vi "JNC Im.vi"(8 "error in (no error)":errorcluster, 10 "Im":u8 format="%04b", 11 "TD4 in":refnum<class "TD4.lvclass">) -> (0 "error out":errorcluster, 3 "TD4 out":refnum<class "TD4.lvclass">)   [LabVIEW 2025, in "TD4.lvclass"]
uses:
  TD4.lvclass
  TD4.lvclass/TD4.ctl
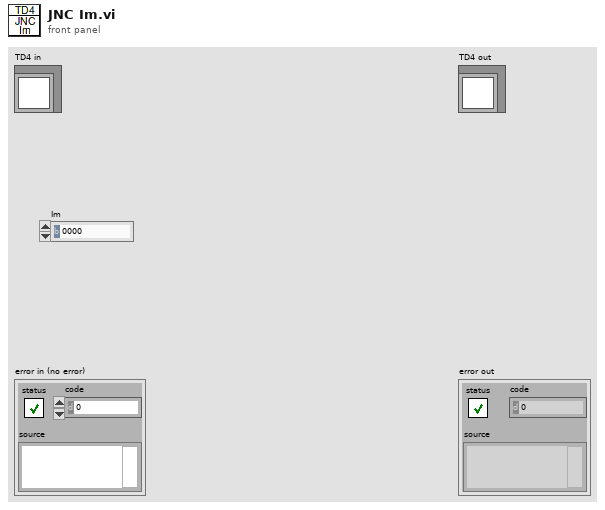
[diagram p1: front panel]
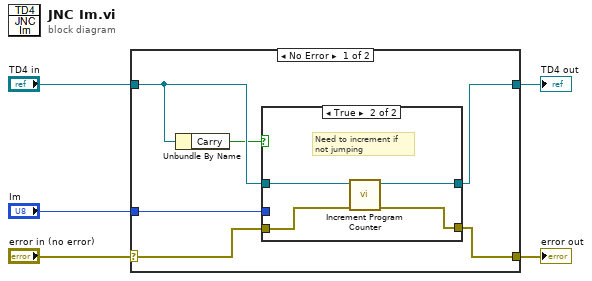
[diagram p0: block diagram]
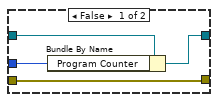
[diagram p2: hidden frame]
diagram:
  n1 = case shown="No Error" "error in (no error)" {
    selector: "error in (no error)" -> [w7 w20]
    tunnel: [w6 w20] -> w4
    tunnel: [w9 w21] -> w2
    tunnel: "TD4 in" -> [w10 w21]
    tunnel: "Im" -> [w11 _]
    frame No Error {
      n2 = Unbundle By Name(w10) -> ("Carry"=w8:bool)
      n3 = case shown="True" w8 {
        tunnel: w11 -> [w15 _]
        tunnel: w10 -> [w14 w19]
        tunnel: [w13 w18] -> w9
        tunnel: w7 -> [w12 w17]
        tunnel: [w12 w16] -> w6
        frame False {
          n4 = Bundle By Name(cluster=w14, "Program Counter"=w15) -> (w13:refnum<class "TD4.lvclass">)
        }
        frame True {
          # "Need to increment if \nnot jumping"
          n5 = call "Increment Program Counter.vi"("error in (no error)"=w17, "TD4 in"=w19) -> ("error out"=w16:errorcluster, "TD4 out"=w18:refnum<class "TD4.lvclass">)  [unwired: 8 in]
        }
      }
    }
    frame Error {
    }
  }
  "error out" <- w4
  "TD4 out" <- w2
